vi "niRFUtil MT UTIL Generate Bits Validate.vi"(0 "Total Bits":i32, 1 "Mode (PN)":T3, 2 "User Base Bit Pattern":T2 min=0, 5 "PN Sequence Order":T4=9, 7 "seed in":T1=3602873842 format="%.0x", 13 "reset?":bool=TRUE) -> (15 "error out":errorcluster)   [LabVIEW 2015, in "niRFUtil.lvlib"]
doc: "This VI validates the inputs for the MT Generate Bits VI."
uses:
  niRFUtil.lvlib
  Includes/niRFUtil INC PN Order.ctl
  Includes/niRFUtil INC Bit Mode.ctl
  Includes/niRFUtil INC Bit Array.ctl
  Includes/niRFUtil INC PN Seed.ctl
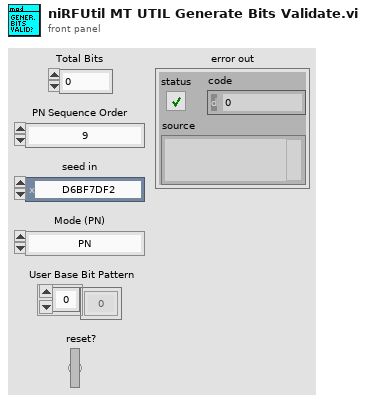
[diagram p1: front panel]
types:
  T1 = typedef "niRFUtil.lvlib/niRFUtil INC PN Seed.ctl" = u32
  T2 = typedef "niRFUtil.lvlib/niRFUtil INC Bit Array.ctl" = i8[]
  T3 = typedef "niRFUtil.lvlib/niRFUtil INC Bit Mode.ctl" = enum16{"PN", "pattern", "user"}
  T4 = typedef "niRFUtil.lvlib/niRFUtil INC PN Order.ctl" = i32
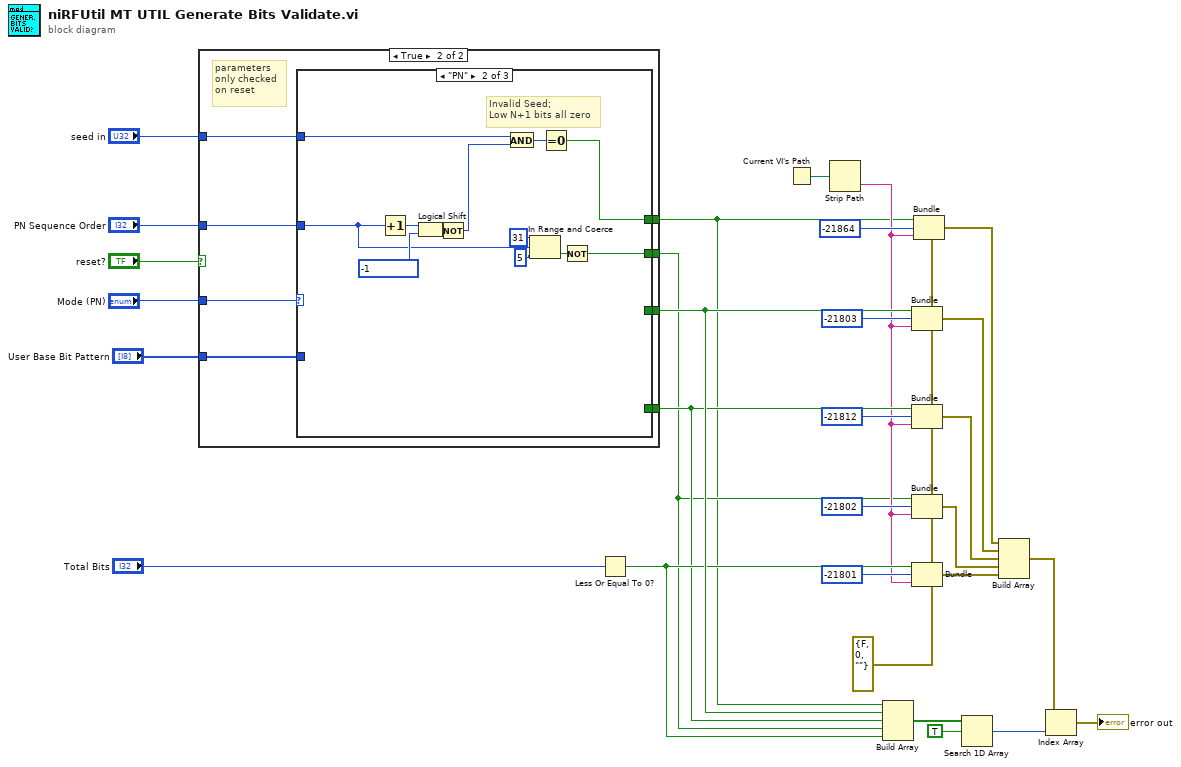
[diagram p0: block diagram]
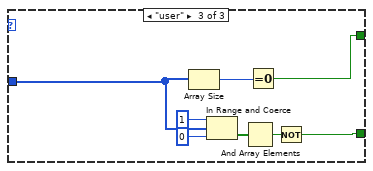
[diagram p4: hidden frame]
diagram:
  w1 = errorcluster {"status"=FALSE, "code"=0, "source"=""} ("error in (no error)")
  n1 = case shown="True" "reset?" {
    tunnel: [_ w37] -> w24
    tunnel: "Mode (PN)" -> [_ w30]
    tunnel: "User Base Bit Pattern" -> [_ w36]
    tunnel: [_ w31] -> w11
    tunnel: [_ w35] -> w7
    tunnel: "PN Sequence Order" -> [_ w34]
    tunnel: "seed in" -> [_ w33]
    tunnel: [_ w32] -> w3
    frame False {
    }
    frame True {
      # "parameters\nonly checked\non reset"
      n2 = case shown="\"PN\"" w30 {
        tunnel: [_ _ w50] -> w37
        tunnel: w36 -> [_ _ w52]
        tunnel: [_ w42 _] -> w35
        tunnel: w34 -> [_ w41 _]
        tunnel: w33 -> [_ w39 _]
        tunnel: [_ w38 _] -> w32
        tunnel: [_ _ w51] -> w31
        frame "pattern", Default {
        }
        frame "PN" {
          # "Invalid Seed;\nLow N+1 bits all zero"
          n3 = Increment(x=w41) -> (x+1=w43:T4)
          n4 = Logical Shift(y=w43, x=-1) -> (x << y=w45:T4)
          n5 = Not(x=w45) -> (.not. x?=w40:T4)
          n6 = And(x=w39, y=w40) -> (x .and. y?=w44:T1)
          n7 = In Range and Coerce(upper limit=31, x=w41, lower limit=5) -> (In Range?=w47:bool)  [unwired: 1 out]
          n8 = Equal To 0?(x=w44) -> (x = 0?=w38:bool)
          n9 = Not(x=w47) -> (.not. x?=w42:bool)
        }
        frame "user" {
          n10 = Array Size(array=w52) -> (size(s)=w57:i32)
          n11 = In Range and Coerce(upper limit=i8 1 ("Numeric"), x=w52, lower limit=i8 0 ("Numeric")) -> (In Range?=w53:bool[])  [unwired: 1 out]
          n12 = And Array Elements(Boolean array=w53) -> (logical AND=w54:bool)
          n13 = Equal To 0?(x=w57) -> (x = 0?=w50:bool)
          n14 = Not(x=w54) -> (.not. x?=w51:bool)
        }
      }
    }
  }
  n15 = Less Or Equal To 0?(x="Total Bits") -> (x <= 0?=w23:bool)
  n16 = Current VI's Path() -> (path=w29:path)
  n17 = Strip Path(path=w29) -> (name=w8:string)  [unwired: 1 out]
  n18 = Build Array(w3, w24, w11, w7, w23) -> (w22:bool[])
  n19 = Bundle(cluster=w1, "status"=w24, "code"=-21803, "source"=w8) -> (w20:errorcluster)
  n20 = Bundle(cluster=w1, "status"=w11, "code"=-21812, "source"=w8) -> (w10:errorcluster)
  n21 = Bundle(cluster=w1, "status"=w7, "code"=-21802, "source"=w8) -> (w19:errorcluster)
  n22 = Bundle(cluster=w1, "status"=w23, "code"=-21801, "source"=w8) -> (w18:errorcluster)
  n23 = Bundle(cluster=w1, "status"=w3, "code"=-21864, "source"=w8) -> (w4:errorcluster)
  n24 = Search 1D Array(1D array=w22, element=TRUE) -> (index of element=w16:i32)  [unwired: 1 out]
  n25 = Build Array(w4, w20, w10, w19, w18) -> (w17:errorcluster[])
  n26 = Index Array(array=w17, index=w16) -> (element=→"error out":errorcluster)
